vi "SpoolLoader.vi"() -> ()   [LabVIEW 2009]
uses:
  Data/GetPixelData16.vi
panel:
  in  "Cycle":bool
  in  "stop":bool
  in  "PixelData":u16[](array[numeric])
  in  "filenames":string[](array[string])
  out "?":u16[][](graph)
  in  "error":errorcluster
  in  "ByteData":u8[](array[numeric])
  in  "AOIStride":i32
  in  "AOIWidth":i32
  in  "AOIHeight":i32
  in  "PixelEncoding":string
  in  "ImageSizeBytes":i32
  in  "Current Image":u32 max=9 step=1
  out "Number of Images":i32
  in  "Path":path
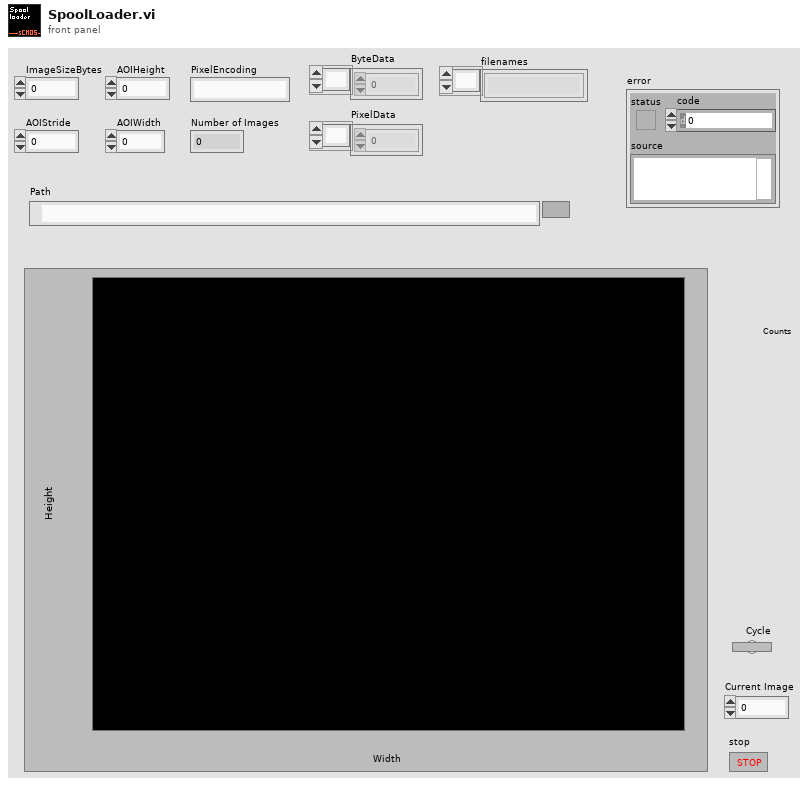
[diagram p1: front panel]
types:
  T1 = enum16{"big-endian, network order", "native, host order", "little-endian"}
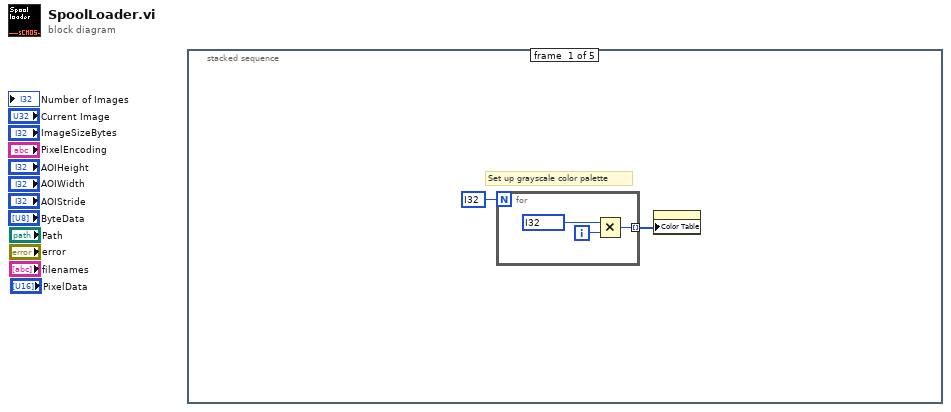
[diagram p0: block diagram]
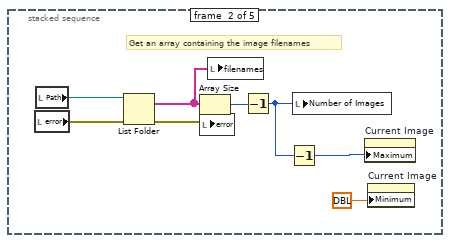
[diagram p2: hidden frame]
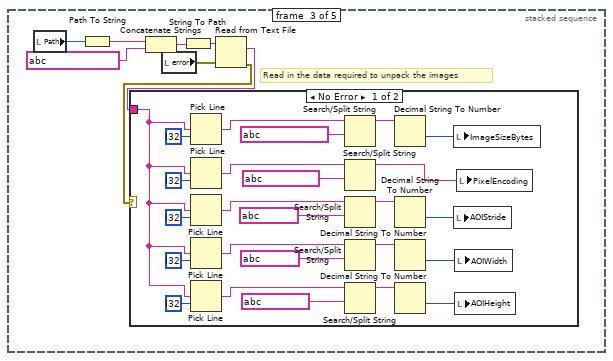
[diagram p3: hidden frame]
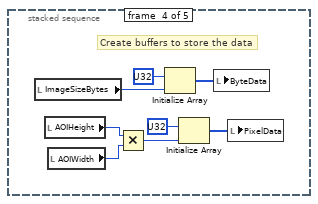
[diagram p5: hidden frame]
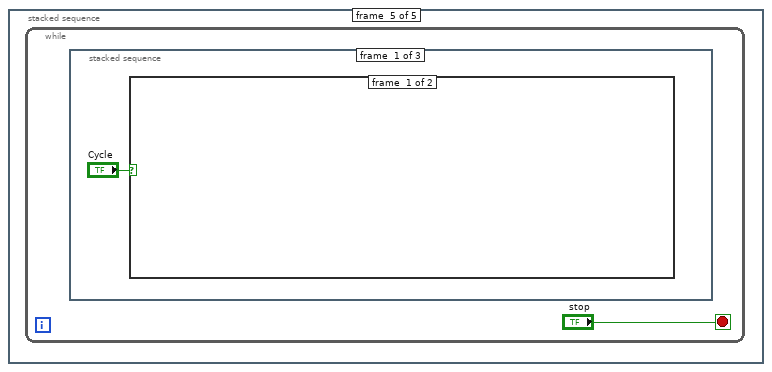
[diagram p6: hidden frame]
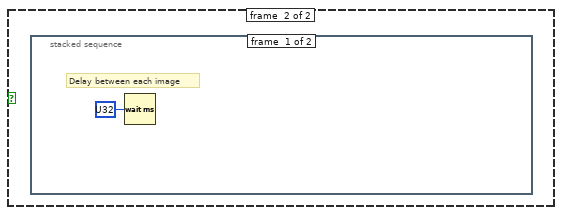
[diagram p7: hidden frame]
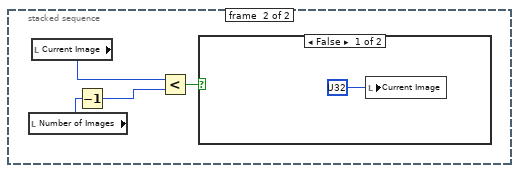
[diagram p8: hidden frame]
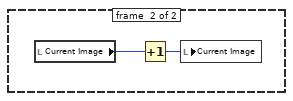
[diagram p9: hidden frame]
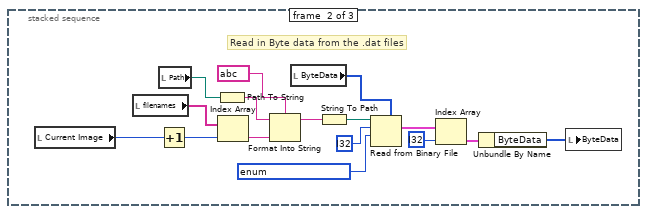
[diagram p10: hidden frame]
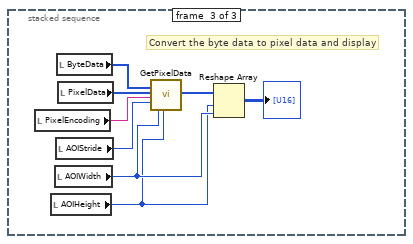
[diagram p11: hidden frame]
diagram:
  n1 = stacked-sequence {
    frame #0 {
      # "Set up grayscale color palette"
      n2 = for {
        N: i32 ? -> [_]
        tunnel: [w3] -> w2 mode=indexing
        i -> [w5]
        n3 = Multiply(x=i32 ?, y=w5) -> (x*y=w3:i32)
      }
      n4 = property class="IntGraph (strict)"("Color Table"=w2) -> ()  [unwired: 2 in, 2 out]
    }
    frame #1 {
      # "Get an array containing the image filenames"
      n5 = local read "error"() -> (w12:errorcluster)
      n6 = local read "Path"() -> (w13:path)
      n7 = List Folder(path=w13, error in=w12) -> (filenames=w10:string[], error out=w11:errorcluster)  [unwired: 2 in, 2 out]
      n8 = Array Size(array=w10) -> (size(s)=w8:i32)
      n9 = local write "error"(w11) -> ()
      n10 = local write "filenames"(w10) -> ()
      n11 = Decrement(x=w8) -> (x-1=w7:i32)
      n12 = Decrement(x=w7) -> (x-1=w6:i32)
      n13 = local write "Number of Images"(w7) -> ()
      n14 = property on="Current Image" class="DigNum (strict)"("Maximum"=w6) -> ()  [unwired: 2 in, 2 out]
      n15 = property on="Current Image" class="DigNum (strict)"("Minimum"=dbl ? ("Data Entry Limits:Minimum")) -> ()  [unwired: 2 in, 2 out]
    }
    frame #2 {
      # "Read in the data required to unpack the images"
      n16 = local read "Path"() -> (w20:path)
      n17 = Path To String(path=w20) -> (string=w18:string)
      n18 = Concatenate Strings(w18, string ? ("format string")) -> (w19:string)
      n19 = local read "error"() -> (w16:errorcluster)
      n20 = String To Path(string=w19) -> (path=w21:path)
      n21 = Read from Text File(file (use dialog)=w21, error in=w16) -> (text=w14:string, error out=w15:errorcluster)  [unwired: 2 in, 2 out]
      n22 = case shown="No Error" w15 {
        tunnel: w14 -> [w22 _]
        frame #0 {
          n23 = Pick Line(multi-line string=w22, line index=i32 ?) -> (output string=w45:string)  [unwired: 1 in]
          n24 = Pick Line(multi-line string=w22, line index=i32 ?) -> (output string=w40:string)  [unwired: 1 in]
          n25 = Pick Line(multi-line string=w22, line index=i32 ?) -> (output string=w24:string)  [unwired: 1 in]
          n26 = Pick Line(multi-line string=w22, line index=i32 ?) -> (output string=w32:string)  [unwired: 1 in]
          n27 = Pick Line(multi-line string=w22, line index=i32 ?) -> (output string=w27:string)  [unwired: 1 in]
          n28 = Search/Split String(string=w45, search string/char (-)=string ?) -> (substring before match=w43:string)  [unwired: 1 in, 2 out]
          n29 = Search/Split String(string=w40, search string/char (-)=string ?) -> (substring before match=w23:string)  [unwired: 1 in, 2 out]
          n30 = Search/Split String(string=w24, search string/char (-)=string ?) -> (substring before match=w25:string)  [unwired: 1 in, 2 out]
          n31 = Search/Split String(string=w32, search string/char (-)=string ?) -> (substring before match=w34:string)  [unwired: 1 in, 2 out]
          n32 = Search/Split String(string=w27, search string/char (-)=string ?) -> (substring before match=w29:string)  [unwired: 1 in, 2 out]
          n33 = Decimal String To Number(string=w43) -> (number=w42:i32)  [unwired: 2 in, 1 out]
          n34 = Decimal String To Number(string=w25) -> (number=w38:i32)  [unwired: 2 in, 1 out]
          n35 = Decimal String To Number(string=w34) -> (number=w35:i32)  [unwired: 2 in, 1 out]
          n36 = Decimal String To Number(string=w29) -> (number=w30:i32)  [unwired: 2 in, 1 out]
          n37 = local write "ImageSizeBytes"(w42) -> ()
          n38 = local write "AOIStride"(w38) -> ()
          n39 = local write "AOIWidth"(w35) -> ()
          n40 = local write "AOIHeight"(w30) -> ()
          n41 = local write "PixelEncoding"(w23) -> ()
        }
        frame #1 {
        }
      }
    }
    frame #3 {
      # "Create buffers to store the data"
      n42 = local read "ImageSizeBytes"() -> (w53:i32)
      n43 = local read "AOIHeight"() -> (w47:i32)
      n44 = local read "AOIWidth"() -> (w48:i32)
      n45 = Multiply(x=w47, y=w48) -> (x*y=w49:i32)
      n46 = Initialize Array(u32 ?, w53) -> (w52:u32[])
      n47 = Initialize Array(u32 ?, w49) -> (w50:u32[])
      n48 = local write "ByteData"(w52) -> ()
      n49 = local write "PixelData"(w50) -> ()
    }
    frame #4 {
      n50 = while {
        stop <- "stop" stop-if-true
        n51 = stacked-sequence {
          frame #0 {
            n52 = case shown="True" "Cycle" {
              frame #0 {
              }
              frame #1 {
                n53 = stacked-sequence {
                  frame #0 {
                    # "Delay between each image"
                    n54 = Wait (ms)(milliseconds to wait=u32 ?) -> ()  [unwired: 1 out]
                  }
                  frame #1 {
                    n55 = local read "Number of Images"() -> (w59:i32)
                    n56 = local read "Current Image"() -> (w61:u32)
                    n57 = Decrement(x=w59) -> (x-1=w58:i32)
                    n58 = Less?(x=w61, y=w58) -> (x < y?=w60:bool)
                    n59 = case shown="False" w60 {
                      frame #0 {
                        n60 = local write "Current Image"(u32 ? ("Current Image")) -> ()
                      }
                      frame #1 {
                        n61 = local read "Current Image"() -> (w64:u32)
                        n62 = Increment(x=w64) -> (x+1=w63:u32)
                        n63 = local write "Current Image"(w63) -> ()
                      }
                    }
                  }
                }
              }
            }
          }
          frame #1 {
            # "Read in Byte data from the .dat files"
            n64 = local read "Current Image"() -> (w80:u32)
            n65 = local read "filenames"() -> (w79:string[])
            n66 = local read "Path"() -> (w68:path)
            n67 = Increment(x=w80) -> (x+1=w72:u32)
            n68 = Path To String(path=w68) -> (string=w67:string)
            n69 = Index Array(array=w79, index=w72) -> (element=w70:string)
            n70 = Format Into String(format string=string ?, initial string=w67, w70) -> (resulting string=w71:string)  [unwired: 1 in, 1 out]
            n71 = local read "ByteData"() -> (w77:u8[])
            n72 = String To Path(string=w71) -> (path=w78:path)
            n73 = Read from Binary File(5:w77, 9:T1 ? ("byte order (0:big-endian, network order)"), 10:i32 ? ("count (1)"), 11:w78) -> (2:w76:cluster{"ByteData":u8[]}[])  [unwired: 2 in, 3 out]
            n74 = Index Array(array=w76, index=i32 ?) -> (element=w74:cluster{"ByteData":u8[]})
            n75 = Unbundle By Name(w74) -> ("ByteData"=w73:u8[])
            n76 = local write "ByteData"(w73) -> ()
          }
          frame #2 {
            # "Convert the byte data to pixel data and display"
            n77 = local read "PixelEncoding"() -> (w87:string)
            n78 = local read "AOIHeight"() -> (w81:i32)
            n79 = local read "AOIWidth"() -> (w82:i32)
            n80 = local read "AOIStride"() -> (w86:i32)
            n81 = local read "ByteData"() -> (w88:u8[])
            n82 = local read "PixelData"() -> (w85:u16[])
            n83 = call-poly "GetPixelData.vi"("Input buffer"=w88, "Output buffer in"=w85, "Pixel Encoding"=w87, "Stride"=w86, "Width"=w82, "Height"=w81) -> ("Output buffer out"=w83:u16[])  [unwired: 11 in, 2 out]
            n84 = Reshape Array(w83, w81, w82) -> (→"?":u16[][])
          }
        }
      }
    }
  }
